vi "XML.InsertChild.vi"(7 "parent":u32, 8 "error in":errorcluster, 10 "name":string, 11 "doc":u32) -> (0 "error out":errorcluster, 2 "new node":u32, 3 "doc out":u32)   [LabVIEW 2019, in "Tools.lvlib"]
uses:
  Tools.lvlib
  LibXML/LibXML.lvlib
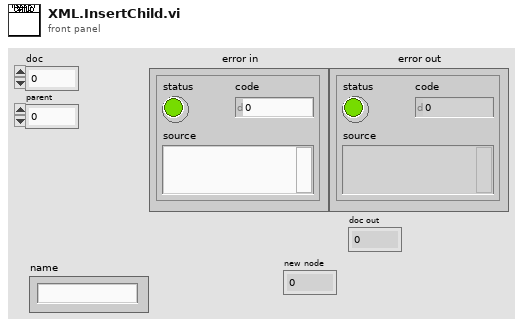
[diagram p1: front panel]
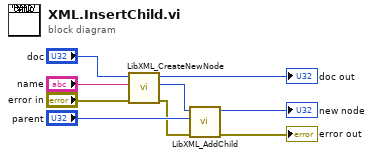
[diagram p0: block diagram]
diagram:
  n1 = call "LibXML_CreateNewNode.vi"("error in"="error in", "name"="name", "doc"="doc") -> ("error out"=w3:errorcluster, "nodePtr out"=w4:u32, "doc out"=→"doc out":u32)  [unwired: 6 in]
  n2 = call "LibXML_AddChild.vi"("error in"=w3, "parent"="parent", "node"=w4) -> ("error out"=→"error out":errorcluster, "node copy"=→"new node":u32)  [unwired: 7 in]
